vi "Disconnect.vi"(8 "error in (no error)":errorcluster, 11 "Serial Device in":refnum<class "Serial Device.lvclass">) -> (0 "error out":errorcluster, 3 "Serial Device out":refnum<class "Serial Device.lvclass">)   [LabVIEW 2017, in "Serial Device.lvclass"]
doc: "Disconnect serial port. It is important to execute this code on exit, so the serial port remains available in subsequent runs."
uses:
  Serial Device.lvclass
  Serial Device.lvclass/Serial Device.ctl
  Get Serial Port.vi
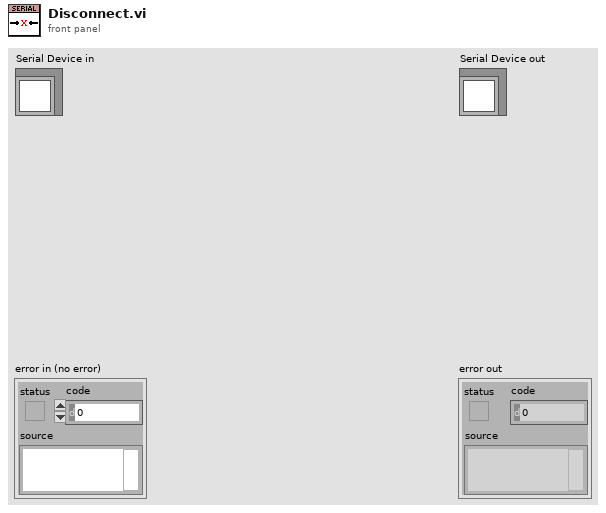
[diagram p1: front panel]
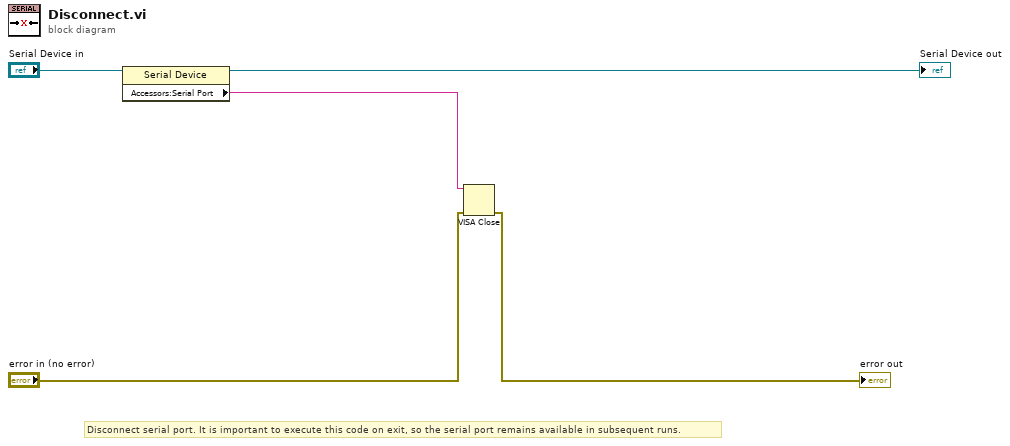
[diagram p0: block diagram]
diagram:
  # "Disconnect serial port. It is important to execute this code on exit, so the serial port remains available in subsequent runs."
  n1 = property class="Serial Device"(reference="Serial Device in") -> (reference out=→"Serial Device out":refnum<class "Serial Device.lvclass">, "Accessors:Serial Port"=w1:string)  [unwired: 1 in, 1 out]
  n2 = VISA Close(VISA resource name=w1, error in (no error)="error in (no error)") -> (error out=→"error out":errorcluster)
